vi "Get Lock.vi"(8 "error in (no error)":errorcluster, 11 "SQLite3LV Connection in":refnum<class "sqlite3.lvclass">) -> (0 "error out":errorcluster, 2 "sqlite lock":refnum<data-value>, 3 "SQLite3LV Connection out":refnum<class "sqlite3.lvclass">)   [LabVIEW 2014, in "SQLite3LV.lvlib" / "sqlite3.lvclass"]
doc: "Returns the lock object associated with the database connection.\n\nClient code is required to implement all synchronization to ensure that the database connection is used by only one thread at a time. \n\nThe helper methods \"Get Lock\" will return a memory reference lock for the database connection. This lock may be use to synchronize access to the database connection from multiple threads or subVIs."
uses:
  sqlite3.lvclass
  sqlite3.lvclass/sqlite3.ctl
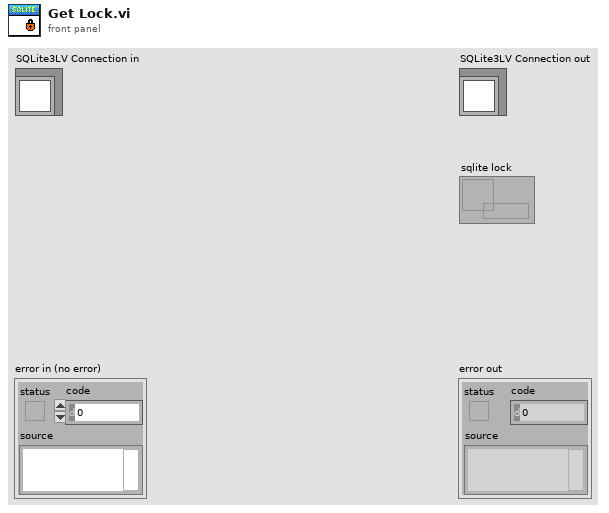
[diagram p1: front panel]
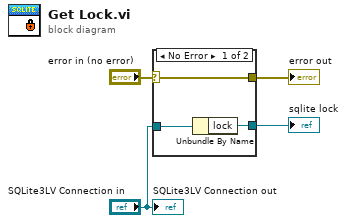
[diagram p0: block diagram]
diagram:
  n1 = case shown="No Error" "error in (no error)" {
    selector: "error in (no error)" -> [w7 w8]
    tunnel: [w7 w8] -> w3
    tunnel: "SQLite3LV Connection in" -> [w6 _]
    tunnel: [w5 _] -> w2
    frame No Error {
      n2 = Unbundle By Name(w6) -> ("lock"=w5:refnum<data-value>)
    }
    frame Error {
    }
  }
  "error out" <- w3
  "sqlite lock" <- w2
  "SQLite3LV Connection out" <- "SQLite3LV Connection in"
